vi "load_hyst_data.vi"(11 "Path":path=path "C:/Users/arnold/Documents/matlab/afm_mpc_journal/unit_tests/labview/hyst_sat_data.csv") -> (0 "h_inv(u_satinv)":dbl[](array[numeric]), 1 "sat_inv(u_nom)":dbl[](array[numeric]), 2 "U_nom":dbl[](array[numeric]), 3 "Cluster":T1, 4 "N_traj":i32)   [LabVIEW 2017, in "Sat_Hyst_TestCase.lvclass"]
uses:
  Sat_Hyst_TestCase.lvclass
  hyst_sat_fxp_16_5_weights.ctl
  <vilib>/Utility/file.llb/Read Delimited Spreadsheet (string).vi
  <vilib>/Utility/file.llb/Read Delimited Spreadsheet (DBL).vi
panel:
  out "all rows 2":string[][](array[string])
  out "all rows":dbl[][](array[numeric])
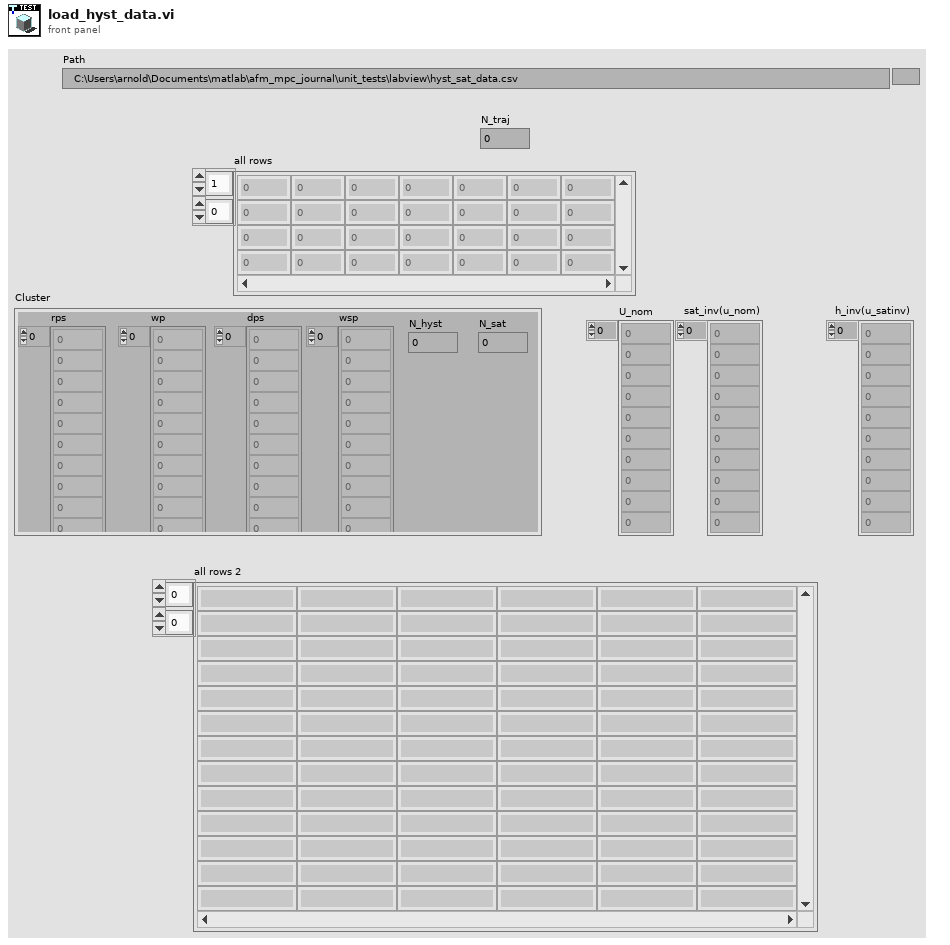
[diagram p1: front panel]
types:
  T1 = typedef "hyst_sat_fxp_16_5_weights.ctl" = cluster{"rps":dbl[], "wp":dbl[], "dps":dbl[], "wsp":dbl[], "N_hyst":i32, "N_sat":i32}
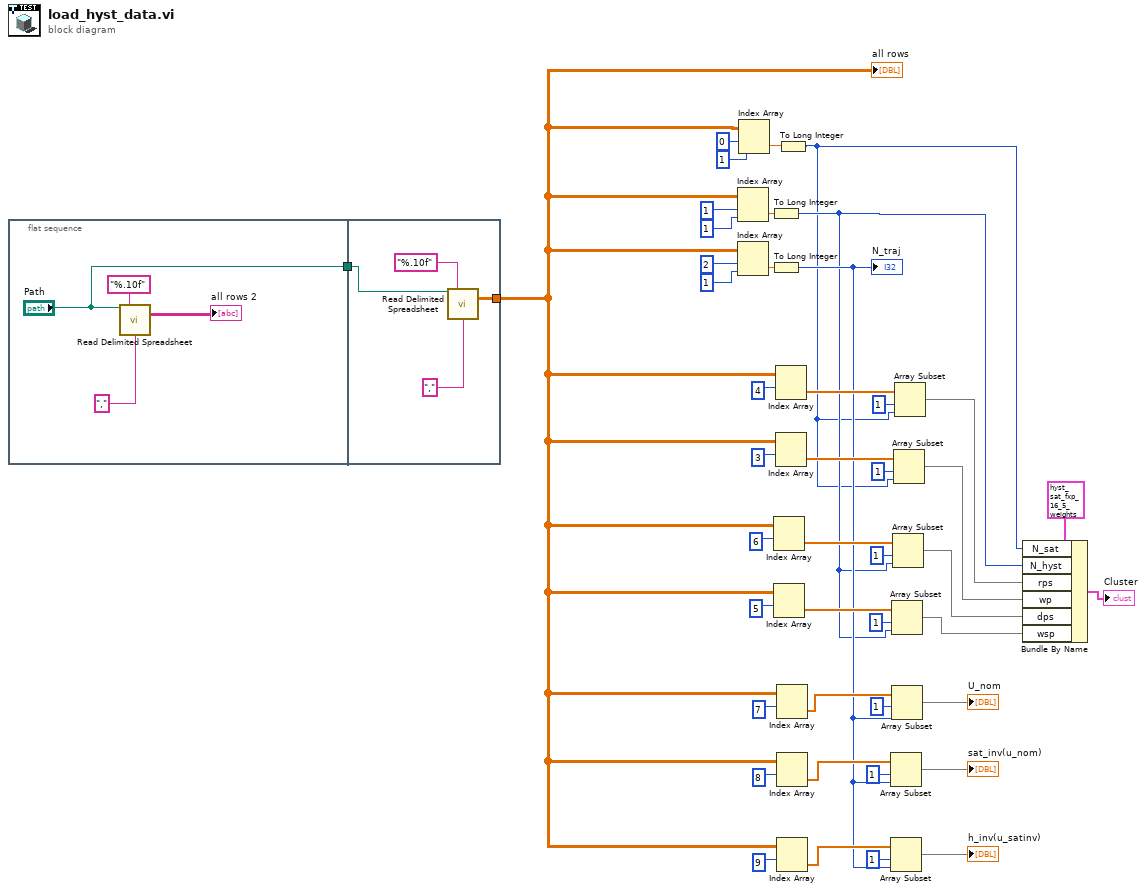
[diagram p0: block diagram]
diagram:
  n1 = flat-sequence {
    tunnel: ["Path"] -> w27
    tunnel: [w50] -> w10
    tunnel: w27 -> [w49]
    frame #0 {
      n2 = call-poly <vilib>:"Read Delimited Spreadsheet.vi"("file path (dialog if empty)"="Path", "format (%s)"="%.10f" ("format (%.3f)"), "delimiter (\\t)"="," ("delimiter (\\t)")) -> ("all rows"=→"all rows 2":string[][])  [unwired: 7 in, 5 out]
    }
    frame #1 {
      n3 = call-poly <vilib>:"Read Delimited Spreadsheet.vi"("file path (dialog if empty)"=w49, "format (%.3f)"="%.10f", "delimiter (\\t)"="," ("delimiter (\\t)")) -> ("all rows"=w50:dbl[][])  [unwired: 7 in, 5 out]
    }
  }
  n4 = Index Array(array=w10, index (row)=1, index (col)=1 ("disabled index (col)")) -> (element=w31:dbl)
  n5 = Index Array(array=w10, index (row)=2, index (col)=1 ("disabled index (col)")) -> (element=w28:dbl)
  n6 = Index Array(array=w10, index (row)=0, index (col)=1 ("disabled index (col)")) -> (element=w37:dbl)
  n7 = To Long Integer(number=w31) -> (32bit integer=w2:i32)
  n8 = To Long Integer(number=w28) -> (32bit integer=w9:i32)
  "N_traj" <- w9
  n9 = Index Array(array=w10, index (row)=6) -> (element=w19:dbl[])  [unwired: 1 in]
  n10 = Index Array(array=w10, index (row)=5) -> (element=w16:dbl[])  [unwired: 1 in]
  n11 = Index Array(array=w10, index (row)=4) -> (element=w42:dbl[])  [unwired: 1 in]
  n12 = Index Array(array=w10, index (row)=3) -> (element=w39:dbl[])  [unwired: 1 in]
  n13 = Index Array(array=w10, index (row)=7) -> (element=w26:dbl[])  [unwired: 1 in]
  n14 = Index Array(array=w10, index (row)=8) -> (element=w25:dbl[])  [unwired: 1 in]
  n15 = Index Array(array=w10, index (row)=9) -> (element=w13:dbl[])  [unwired: 1 in]
  n16 = To Long Integer(number=w37) -> (32bit integer=w1:i32)
  n17 = Array Subset(array=w25, index=1, length=w9) -> (→"sat_inv(u_nom)":dbl[])
  n18 = Array Subset(array=w13, index=1, length=w9) -> (→"h_inv(u_satinv)":dbl[])
  n19 = Array Subset(array=w16, index=1, length=w2) -> (w3:dbl[])
  n20 = Array Subset(array=w26, index=1, length=w9) -> (→"U_nom":dbl[])
  n21 = Array Subset(array=w19, index=1, length=w2) -> (w4:dbl[])
  n22 = Array Subset(array=w39, index=1, length=w1) -> (w5:dbl[])
  n23 = Array Subset(array=w42, index=1, length=w1) -> (w6:dbl[])
  n24 = Bundle By Name(cluster=T1 {"rps"=[0.0, 0.956055, 2.098145, 3.352051, 4.671875, 6.046875, 7.470703], "wp"=[1.379395, -0.225098, -0.103027, -0.052734, -0.040039, -0.032715, -0.059082], "dps"=[-9.0, -5.399902, -1.799805, 0.0, 1.799805, 5.399902, 9.0], "wsp"=[0.006836, -0.039551, -0.038086, 0.736328, 0.045898, 0.072754, 0.072266], "N_hyst"=7, "N_sat"=7} ("Cluster 2"), "N_sat"=w1, "N_hyst"=w2, "rps"=w6, "wp"=w5, "dps"=w4, "wsp"=w3) -> (→"Cluster":T1)
  "all rows" <- w10
